vi "Round2_10th.vi"(11 "Newman":dbl format="%#.7g") -> (3 "Newmout":dbl)   [LabVIEW 2015]
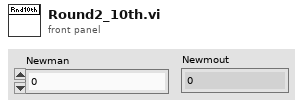
[diagram p1: front panel]
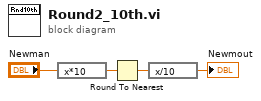
[diagram p0: block diagram]
diagram:
  n1 = expression code="x*10"("Newman") -> (w3:dbl)
  n2 = Round To Nearest(number=w3) -> (nearest integer value=w2:dbl)
  n3 = expression code="x/10"(w2) -> (→"Newmout":dbl)
